vi "Clear Subset.vi"(8 "error in (no error)":errorcluster, 9 "offset (0)":u64 format="%d bytes", 10 "length (-1: rest)":i64=-1 format="%d bytes", 11 "Pointer in":refnum<class "Pointer.lvclass">) -> (0 "error out":errorcluster, 3 "Pointer out":refnum<class "Pointer.lvclass">)   [LabVIEW 2016, in "Memory Manager.lvlib" / "Pointer.lvclass"]
doc: "Sets the subset of bytes specified by <b>offset</b> and <b>length</b> within the provided <b>pointer</b> to zero.\n\n<b>Note:</b> This VI is <b>safe</b>, meaning it performs null pointer and bounds checks to prevent invaid memory access."
uses:
  Pointer.lvclass
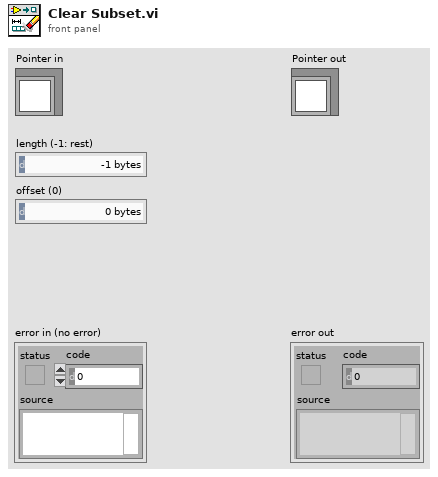
[diagram p1: front panel]
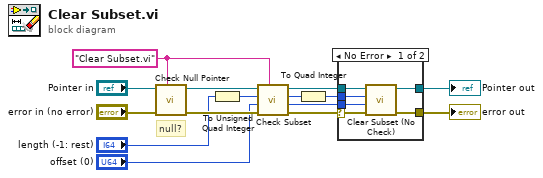
[diagram p0: block diagram]
diagram:
  w11 = "Clear Subset.vi" ("source vi name")
  # "null?"
  n1 = call "Check Null Pointer.vi"("source vi name"=w11, "error in (no error)"="error in (no error)", "Pointer in"="Pointer in") -> ("error out"=w15:errorcluster, "Pointer out"=w4:refnum<class "Pointer.lvclass">)  [unwired: 7 in]
  n2 = To Unsigned Quad Integer(1:"length (-1: rest)") -> (0:w3:u64)
  n3 = call "Check Subset.vi"("source vi name"=w11, "error in (no error)"=w15, "offset (0)"="offset (0)", "length"=w3, "Pointer in"=w4) -> ("error out"=w5:errorcluster, "offset out"=w8:u64, "length"=w9:u64, "Pointer out"=w10:refnum<class "Pointer.lvclass">)  [unwired: 3 in]
  n4 = To Quad Integer(1:w9) -> (0:w2:i64)
  n5 = case shown="No Error" w5 {
    selector: w5 -> [w16 w22]
    tunnel: w10 -> [w21 w23]
    tunnel: w2 -> [w20 _]
    tunnel: w8 -> [w19 _]
    tunnel: [w18 w23] -> w7
    tunnel: [w17 w22] -> w6
    frame No Error {
      n6 = call "Clear Subset (No Check).vi"("error in (no error)"=w16, "offset (0)"=w19, "length (-1: rest)"=w20, "Pointer in"=w21) -> ("error out"=w17:errorcluster, "Pointer out"=w18:refnum<class "Pointer.lvclass">)  [unwired: 6 in]
    }
    frame Error {
    }
  }
  "error out" <- w6
  "Pointer out" <- w7
